vi "Create Channel Task.vi"(8 "error in":errorcluster, 10 "SQL query":string="SELECT max(MaximumVoltage),max(MinimumVoltage), max(TerminalConfiguration),max(SampleRate) FROM ltt.daq_configuration \nWhere ChannelType='Analog_Output' and Enabled=1;", 11 "NI Analog Output in":refnum<class "NI Analog Output.lvclass">) -> (0 "error out":errorcluster, 3 "NI Analog Output out":refnum<class "NI Analog Output.lvclass">)   [LabVIEW 2023, in "HardwareAbstractionLayer_LVOOP.lvlib" / "NI Analog Output.lvclass"]
doc: "This VI Analog Output Physical Channel Based DAQmx Create Channel"
uses:
  NI Analog Output.lvclass
  NI Analog Output.lvclass/NI Analog Output.ctl
  <vilib>/DAQmx/create/channels.llb/DAQmx Create Channel (AO-Voltage-Basic).vi
  <vilib>/DAQmx/configure/timing.llb/DAQmx Timing (Sample Clock).vi
  Database/Database.lvclass
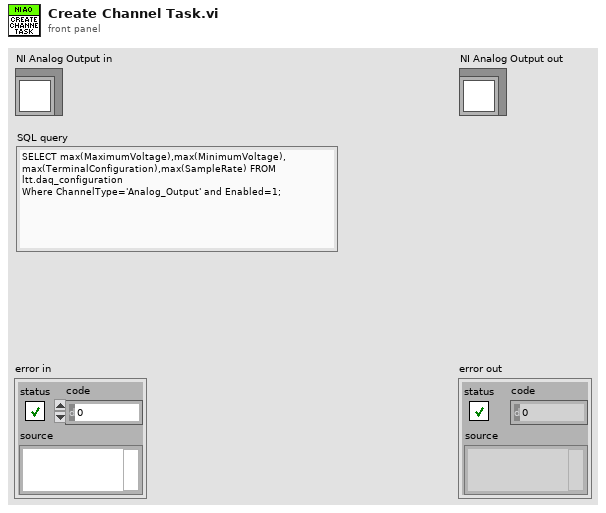
[diagram p1: front panel]
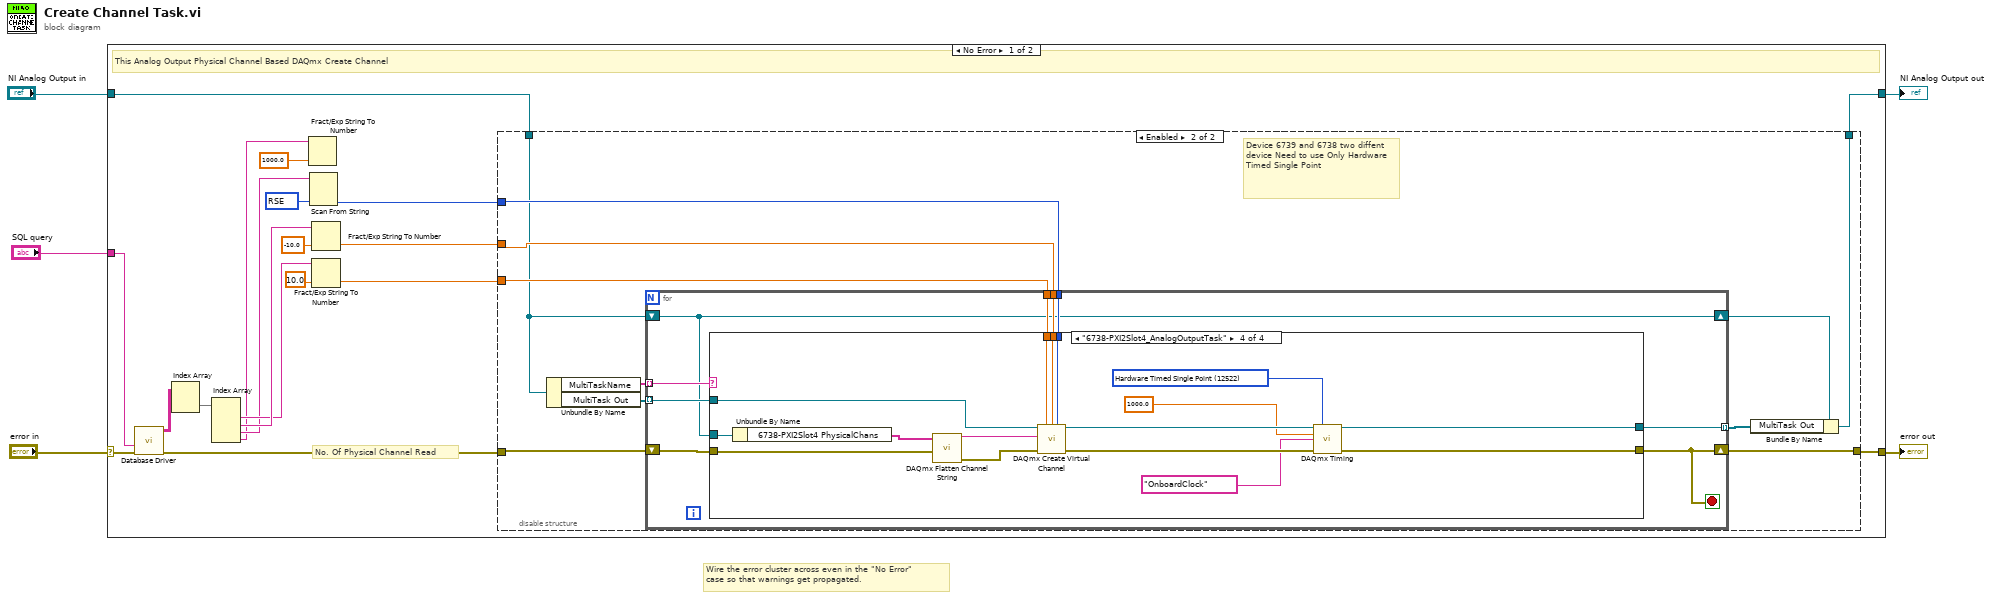
[diagram p0: block diagram]
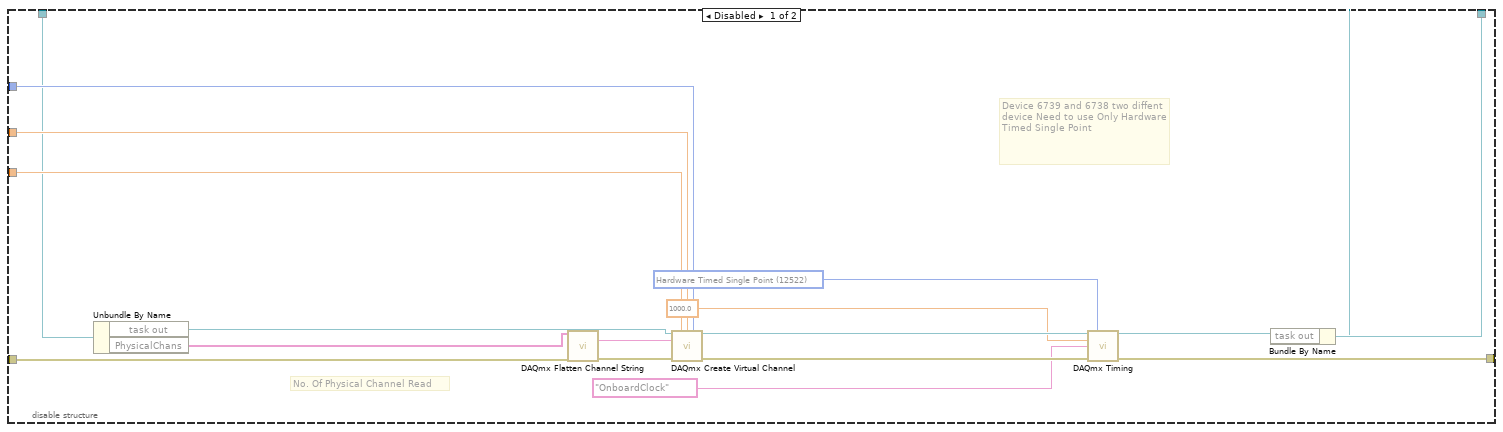
[diagram p2: hidden frame]
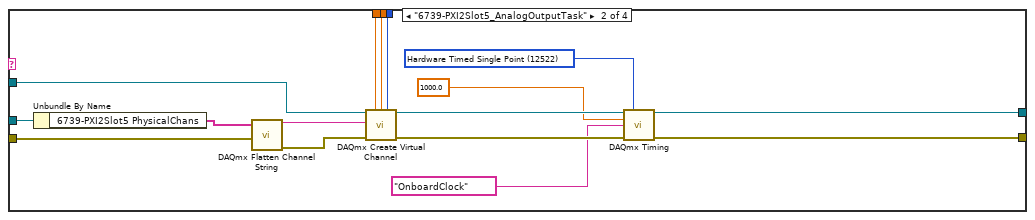
[diagram p4: hidden frame]
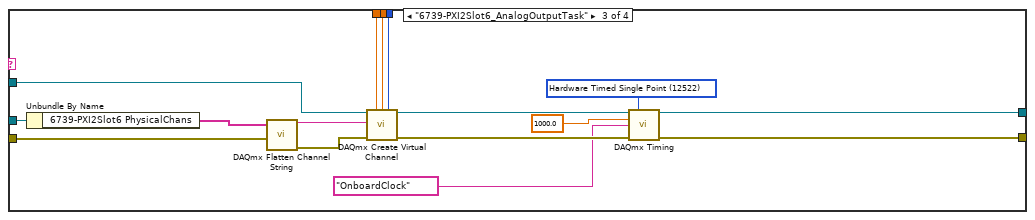
[diagram p5: hidden frame]
diagram:
  # "Wire the error cluster across even in the \"No Error\"\ncase so that warnings get propagated."
  n1 = case shown="No Error" "error in" {
    selector: "error in" -> [w9 w112]
    tunnel: [w6 w112] -> w4
    tunnel: [w12 w111] -> w2
    tunnel: "NI Analog Output in" -> [w11 w111]
    tunnel: "SQL query" -> [w7 _]
    frame No Error {
      w21 = 10083 items=["Default"=-1, "RSE"=10083, "NRSE"=10078, "Differential"=10106, "Pseudodifferential"=12529] ("input terminal configuration")
      # "No. Of Physical Channel Read"
      # "This Analog Output Physical Channel Based DAQmx Create Channel"
      n2 = call "Database Driver.vi"("error in"=w9, "SQL query"=w7) -> ("error out"=w8:errorcluster, "data"=w10:string[][])  [unwired: 6 in, 2 out]
      n3 = Index Array(array=w10) -> (element=w22:string[])  [unwired: 2 in]
      n4 = Index Array(array=w22) -> (element #1=w23:string, element #2=w24:string, element #3=w15:string, element #4=w13:string)  [unwired: 4 in]
      n5 = Fract/Exp String To Number(string=w13, default (0 dbl)=1000.0 ("rate")) -> ()  [unwired: 2 in, 2 out]
      n6 = Scan From String(input string=w15, default 1=w21) -> (output 1=w16:i32)  [unwired: 3 in, 3 out]
      n7 = Fract/Exp String To Number(string=w24, default (0 dbl)=-10.0 ("maximum value")) -> (number=w17:dbl)  [unwired: 2 in, 1 out]
      n8 = Fract/Exp String To Number(string=w23, default (0 dbl)=10.0 ("maximum value")) -> (number=w18:dbl)  [unwired: 2 in, 1 out]
      n9 = disable-structure shown="Enabled" {
        disable-tunnel: w18 -> [w41 w48]
        disable-tunnel: w17 -> [w40 w49]
        disable-tunnel: w16 -> [w39 w50]
        disable-tunnel: [w34 w42] -> w12
        disable-tunnel: w11 -> [w33 w46]
        disable-tunnel: w8 -> [w32 w52]
        disable-tunnel: [w29 w51] -> w6
        frame Disabled {
          w25 = 12522 items=["Finite Samples"=10178, "Continuous Samples"=10123, "Hardware Timed Single Point"=12522] ("sample mode")
          # "Device 6739 and 6738 two diffent device Need to use Only Hardware Timed Single Point"
          # "No. Of Physical Channel Read"
          n10 = Unbundle By Name(w33) -> ("task out"=w35:refnum<k21>, "PhysicalChans"=w37:tag[])
          n11 = call <vilib>:"DAQmx Flatten Channel String.vi"("names in"=w37, "error in"=w32) -> ("names out"=w36:string, "error out"=w38:errorcluster)  [unwired: 12 in]
          n12 = call-poly <vilib>:"DAQmx Create Virtual Channel.vi"("task in"=w35, "maximum value"=w41, "minimum value"=w40, "output terminal configuration"=w39, "physical channels"=w36, "error in"=w38) -> ("task out"=w31:refnum<k21>, "error out"=w28:errorcluster)  [unwired: 8 in]
          n13 = call-poly <vilib>:"DAQmx Timing.vi"("task/channels in"=w31, "sample mode"=w25, "rate"=1000.0, "source"=tag "OnboardClock", "error in"=w28) -> ("task out"=w30:refnum<k21>, "error out"=w29:errorcluster)  [unwired: 9 in]
          n14 = Bundle By Name(cluster=w33, "task out"=w30) -> (w34:refnum<class "NI Analog Output.lvclass">)
        }
        frame Enabled {
          # "Device 6739 and 6738 two diffent device Need to use Only Hardware Timed Single Point"
          n15 = Unbundle By Name(w46) -> ("MultiTaskName"=w47:string[], "MultiTask Out"=w45:refnum<k21>[])
          n16 = for {
            tunnel: w50 -> [w60]
            tunnel: w49 -> [w59]
            tunnel: w48 -> [w58]
            shift-right: [w53] -> w51
            shift-left: w52 -> [w61]
            tunnel: w47 -> [w57] mode=indexing
            shift-right: [w55] -> w44
            shift-left: w46 -> [w55]
            tunnel: w45 -> [w56] mode=indexing
            tunnel: [w54] -> w43 mode=indexing
            stop <- w53 stop-if-true
            n17 = case shown="\"6738-PXI2Slot4_AnalogOutputTask\"" w57 {
              tunnel: w61 -> [w62 w71 w94 w103]
              tunnel: [w62 w70 w93 w102] -> w53
              tunnel: w60 -> [_ w69 w92 w101]
              tunnel: w59 -> [_ w68 w91 w100]
              tunnel: w58 -> [_ w67 w90 w99]
              tunnel: w55 -> [_ w66 w89 w98]
              tunnel: w56 -> [_ w64 w87 w96]
              tunnel: [_ w63 w86 w95] -> w54
              frame "", Default {
              }
              frame "6739-PXI2Slot5_AnalogOutputTask" {
                w72 = 12522 items=["Finite Samples"=10178, "Continuous Samples"=10123, "Hardware Timed Single Point"=12522] ("sample mode")
                n18 = Unbundle By Name(w66) -> ("6739-PXI2Slot5 PhysicalChans"=w65:tag[])
                n19 = call <vilib>:"DAQmx Flatten Channel String.vi"("names in"=w65, "error in"=w71) -> ("names out"=w77:string, "error out"=w78:errorcluster)  [unwired: 12 in]
                n20 = call-poly <vilib>:"DAQmx Create Virtual Channel.vi"("task in"=w64, "maximum value"=w67, "minimum value"=w68, "output terminal configuration"=w69, "physical channels"=w77, "error in"=w78) -> ("task out"=w76:refnum<k21>, "error out"=w75:errorcluster)  [unwired: 8 in]
                n21 = call-poly <vilib>:"DAQmx Timing.vi"("task/channels in"=w76, "sample mode"=w72, "rate"=1000.0, "source"=tag "OnboardClock", "error in"=w75) -> ("task out"=w63:refnum<k21>, "error out"=w70:errorcluster)  [unwired: 9 in]
              }
              frame "6739-PXI2Slot6_AnalogOutputTask" {
                w79 = 12522 items=["Finite Samples"=10178, "Continuous Samples"=10123, "Hardware Timed Single Point"=12522] ("sample mode")
                n22 = Unbundle By Name(w89) -> ("6739-PXI2Slot6 PhysicalChans"=w88:tag[])
                n23 = call <vilib>:"DAQmx Flatten Channel String.vi"("names in"=w88, "error in"=w94) -> ("names out"=w84:string, "error out"=w85:errorcluster)  [unwired: 12 in]
                n24 = call-poly <vilib>:"DAQmx Create Virtual Channel.vi"("task in"=w87, "maximum value"=w90, "minimum value"=w91, "output terminal configuration"=w92, "physical channels"=w84, "error in"=w85) -> ("task out"=w83:refnum<k21>, "error out"=w82:errorcluster)  [unwired: 8 in]
                n25 = call-poly <vilib>:"DAQmx Timing.vi"("task/channels in"=w83, "sample mode"=w79, "rate"=1000.0, "source"=tag "OnboardClock", "error in"=w82) -> ("task out"=w86:refnum<k21>, "error out"=w93:errorcluster)  [unwired: 9 in]
              }
              frame "6738-PXI2Slot4_AnalogOutputTask" {
                w104 = 12522 items=["Finite Samples"=10178, "Continuous Samples"=10123, "Hardware Timed Single Point"=12522] ("sample mode")
                n26 = Unbundle By Name(w98) -> ("6738-PXI2Slot4 PhysicalChans"=w97:tag[])
                n27 = call <vilib>:"DAQmx Flatten Channel String.vi"("names in"=w97, "error in"=w103) -> ("names out"=w109:string, "error out"=w110:errorcluster)  [unwired: 12 in]
                n28 = call-poly <vilib>:"DAQmx Create Virtual Channel.vi"("task in"=w96, "maximum value"=w99, "minimum value"=w100, "output terminal configuration"=w101, "physical channels"=w109, "error in"=w110) -> ("task out"=w108:refnum<k21>, "error out"=w107:errorcluster)  [unwired: 8 in]
                n29 = call-poly <vilib>:"DAQmx Timing.vi"("task/channels in"=w108, "sample mode"=w104, "rate"=1000.0, "source"=tag "OnboardClock", "error in"=w107) -> ("task out"=w95:refnum<k21>, "error out"=w102:errorcluster)  [unwired: 9 in]
              }
            }
          }
          n30 = Bundle By Name(cluster=w44, "MultiTask Out"=w43) -> (w42:refnum<class "NI Analog Output.lvclass">)
        }
      }
    }
    frame Error {
    }
  }
  "error out" <- w4
  "NI Analog Output out" <- w2
